vi "FolderPath.vi"(8 "error in":errorcluster caption="错误输入", 9 "FolerName":string, 11 "PathIn":path) -> (0 "error out":errorcluster caption="错误输出", 3 "PathOut":path)   [LabVIEW 2013]
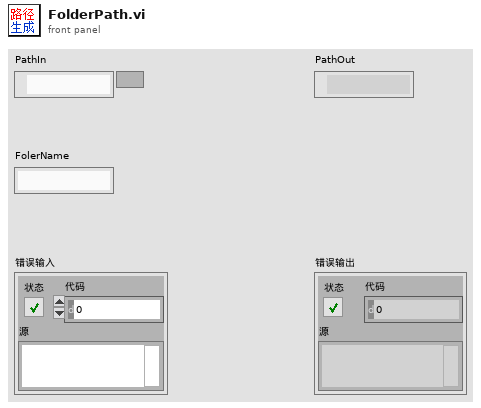
[diagram p1: front panel]
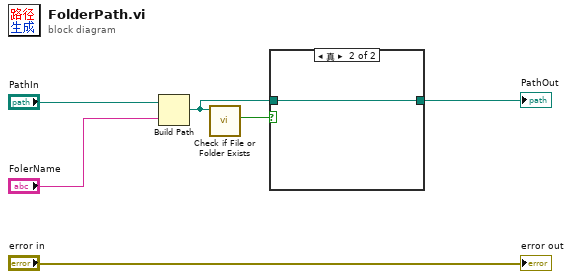
[diagram p0: block diagram]
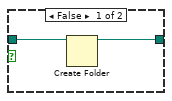
[diagram p2: hidden frame]
diagram:
  n1 = Build Path(base path="PathIn", name or relative path="FolerName") -> (appended path=w2:path)
  n2 = call <vilib>:"Check if File or Folder Exists.vi"("path"=w2) -> ("file or folder exists?"=w4:bool)  [unwired: 8 in, 2 out]
  n3 = case shown="真" w4 {
    tunnel: [w7 w9] -> w3
    tunnel: w2 -> [w8 w9]
    frame False {
      n4 = Create Folder(path (use dialog)=w8) -> (created path=w7:path)  [unwired: 2 in, 2 out]
    }
    frame True {
    }
  }
  "PathOut" <- w3
  "error out" <- "error in"
